vi "U6 easy Stream.vi"() -> ()   [LabVIEW 2020]
panel:
  out "Data":dbl[][](array[numeric]) format="%.3f"
  out "Waveform Graph":dbl[][](graph)
  in  "Scan List (+)":u8[](array[numeric])=[0, 1, 2, 3]
  out "# of iterations":i32
  in  "Scan Rate (Hz)":dbl=1000.0 format="%.3f"
  in  "stop":bool
  out "Error Message":string
  # "This example streams from the first found USB U6."
  # "The + scan list is the positive\nchannels.  This example will just\nuse 199 for negative channels\nmeaning single-ended.\n\nTo remove an element, right-click\non it, select Data Operations =>\nRemove Element.\n\nTo empty an array, right-click\nnear the edge, select Data\nOperations => Empty Array.\n\nOther useful operations:  From the\nOperate menu are \"Make Current\nValues Default\" and \"Reinitialize\nTo Default\"."
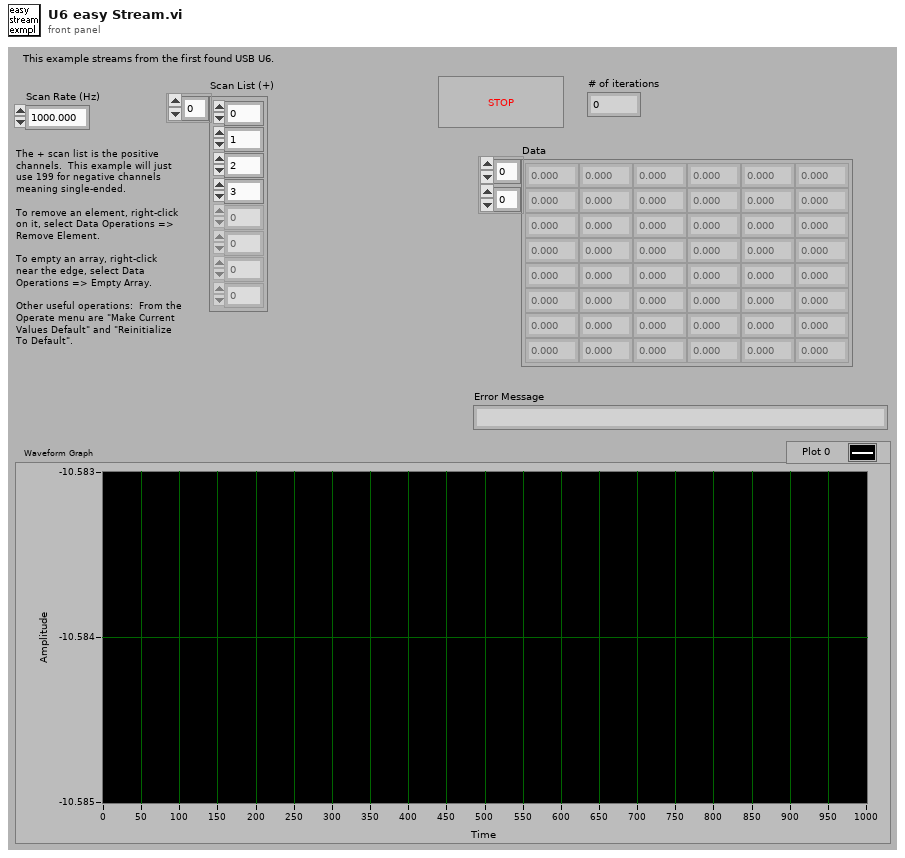
[diagram p1: front panel]
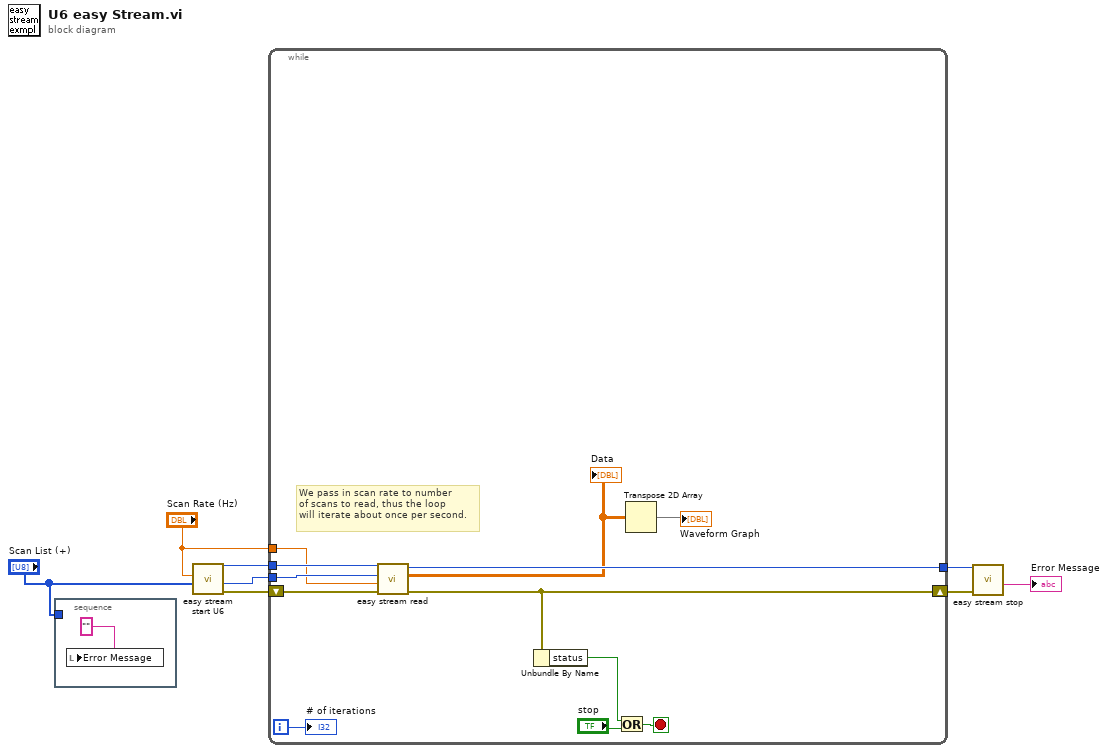
[diagram p0: block diagram]
diagram:
  n1 = stacked-sequence {
    tunnel: "Scan List (+)" -> [_]
    frame #0 {
      n2 = local write "Error Message"("" ("Error Message")) -> ()
    }
  }
  n3 = call "easy stream start U6.vi"("Scan List (+)"="Scan List (+)", "Scan Rate (Hz)"="Scan Rate (Hz)") -> ("error out"=w2:errorcluster, "# Channels"=w8:i32, "Handle Out"=w7:i32)  [unwired: 6 in, 1 out]
  n4 = while {
    tunnel: "Scan Rate (Hz)" -> [w10]
    tunnel: [w13] -> w5
    tunnel: w7 -> [w14]
    tunnel: w8 -> [w15]
    shift-left: w2 -> [w16]
    shift-right: [w11] -> w6
    i -> [w18]
    stop <- w19 stop-if-true
    # "We pass in scan rate to number\nof scans to read, thus the loop\nwill iterate about once per second."
    n5 = call "easy stream read.vi"("error in"=w16, "Scans To Read"=w10, "# Channels In Stream"=w15, "Handle In"=w14) -> ("error out"=w11:errorcluster, "Data"=w12:dbl[][], "Handle Out"=w13:i32)  [unwired: 4 in, 1 out]
    "Data" <- w12
    n6 = Unbundle By Name(w11) -> ("status"=w20:bool)
    n7 = Or(x=w20, y="stop") -> (x .or. y?=w19:bool)
    n8 = Transpose 2D Array(2D array=w12) -> (transposed array=→"Waveform Graph":dbl[][])
    "# of iterations" <- w18
  }
  n9 = call "easy stream stop.vi"("error in"=w6, "Handle In"=w5) -> ("Error Message"=→"Error Message":string)  [unwired: 7 in, 2 out]
